vi "Red Pitaya Control.vi"(8 "Error In":errorcluster, 10 "Server port":u16=1002, 11 "Server address":string="192.168.1.100") -> (0 "Error Out":errorcluster)   [LabVIEW 2016]
uses:
  Mode.ctl
  Red Pitaya Parameters.ctl
  Waform generation/I-V parameters.ctl
  RP Command.ctl
  RP Config Offsets.ctl
  RP Write Command TCP.vi
  RP Read Temperature TCP.vi
  RP Read Status TCP.vi
  RP Read Subset TCP.vi
panel:
  in  "I-V parameters":T1={"Start magnitude"=0.001, "Magnitude increment"=0.001, "Number of pulses"=7, "Baseline length"=480, "Ramp length"=32, "Top  length"=480, "Threshold "=0.0001, "Processing delay"=255, "Valhalla range"=0.01, "Interpolation"=64} {"Valhalla range" format="%#_6pA"; "Processing delay" format="%dpts"; "Threshold" format="%#_6pV"; "Top  length" format="%dpts"; "Ramp length" format="%dpts"; "Baseline length" format="%dpts"; "Magnitude increment" format="%#_6pA"; "Start magnitude" format="%#_6pA"}
  in  "no bram":bool
  out "Output Waveform":i16[](graph)
  in  "Write waveform":bool
  in  "Controls":enum32{"Basic", "Advanced"}(tab)
  out "X&Y":cluster{i32, i32}(graph)
  in  "Parameters":T2={"Ranges"=[0.01, 0.01], "Output frequency 1"=15625000.0, "Output frequency 2"=50000.0, "Pre-trigger samples"=600000, "Post-trigger samples"=11534336, "Desimation rate"=1, "Delayed start"=571428} {"Delayed start" format="0x%x (%d)"; "Post-trigger samples" format="0x%x (%d)"; "Pre-trigger samples" format="0x%x (%d)"; "Output frequency 2" format="%#_6p"; "Output frequency 1" format="%#_6p"; "Ranges" format="%#_12p"}
  out "CPU Temperature":dbl(slide)=48.847186279148 scale=0.0..100.0
  out "Y":i32=1717987 format="0x%x (%d)"
  out "X":i32=1717987 format="0x%x (%d)"
  in  "Read XY":bool
  in  "Trigger pos acuracy":i32=1
  in  "Signal bits":i32=14
  in  "Read Temperature":bool
  in  "Read trigger":bool=TRUE
  in  "Start server":bool
  in  "FPGA Logic":enum16{"Digitizer", "Fast Digitizer"}(ring)
  in  "Auto-save file":bool
  in  "Samples to read":u64=67108864 format="0x%x (%d)"
  in  "Record":bool
  out "Server  output":string
  out "Temperature Chart":dbl(graph)=48.847186279148
  out "bytes written":i32=8
  in  "Status":bool
  out "Status response":u32=4294967115 format="0x%x (%d)"
  out "element":u32
  in  "Status offset":u64=12
  out "Record start pos":u32=20519343
  out "x-y":u32=181
  out "Phase increment 2":u64=1717987
  out "Phase increment 1":u64=1717987 format="0x%x (%d)"
  in  "Process Stop Button":bool
  in  "Read":bool
  in  "Baseline start":u16=255
  in  "Send \"Connect client\"":bool=TRUE
  out "sts bits":u32=3 format="%07b"
  in  "Read subset":bool
  out "Data File  Path":path=path "C:/Data/January_2017/011017/rp194452_011017.tdms"
  out "Trigger state":bool
  in  "Trigger":bool
  in  "Arm":bool
  out "Phase  Graph":u32[](graph)
  in  "Mode":T3=enum."Current-Voltage"
  out "Waveform Graph":sgl[][](graph)
  in  "Stop Server":bool
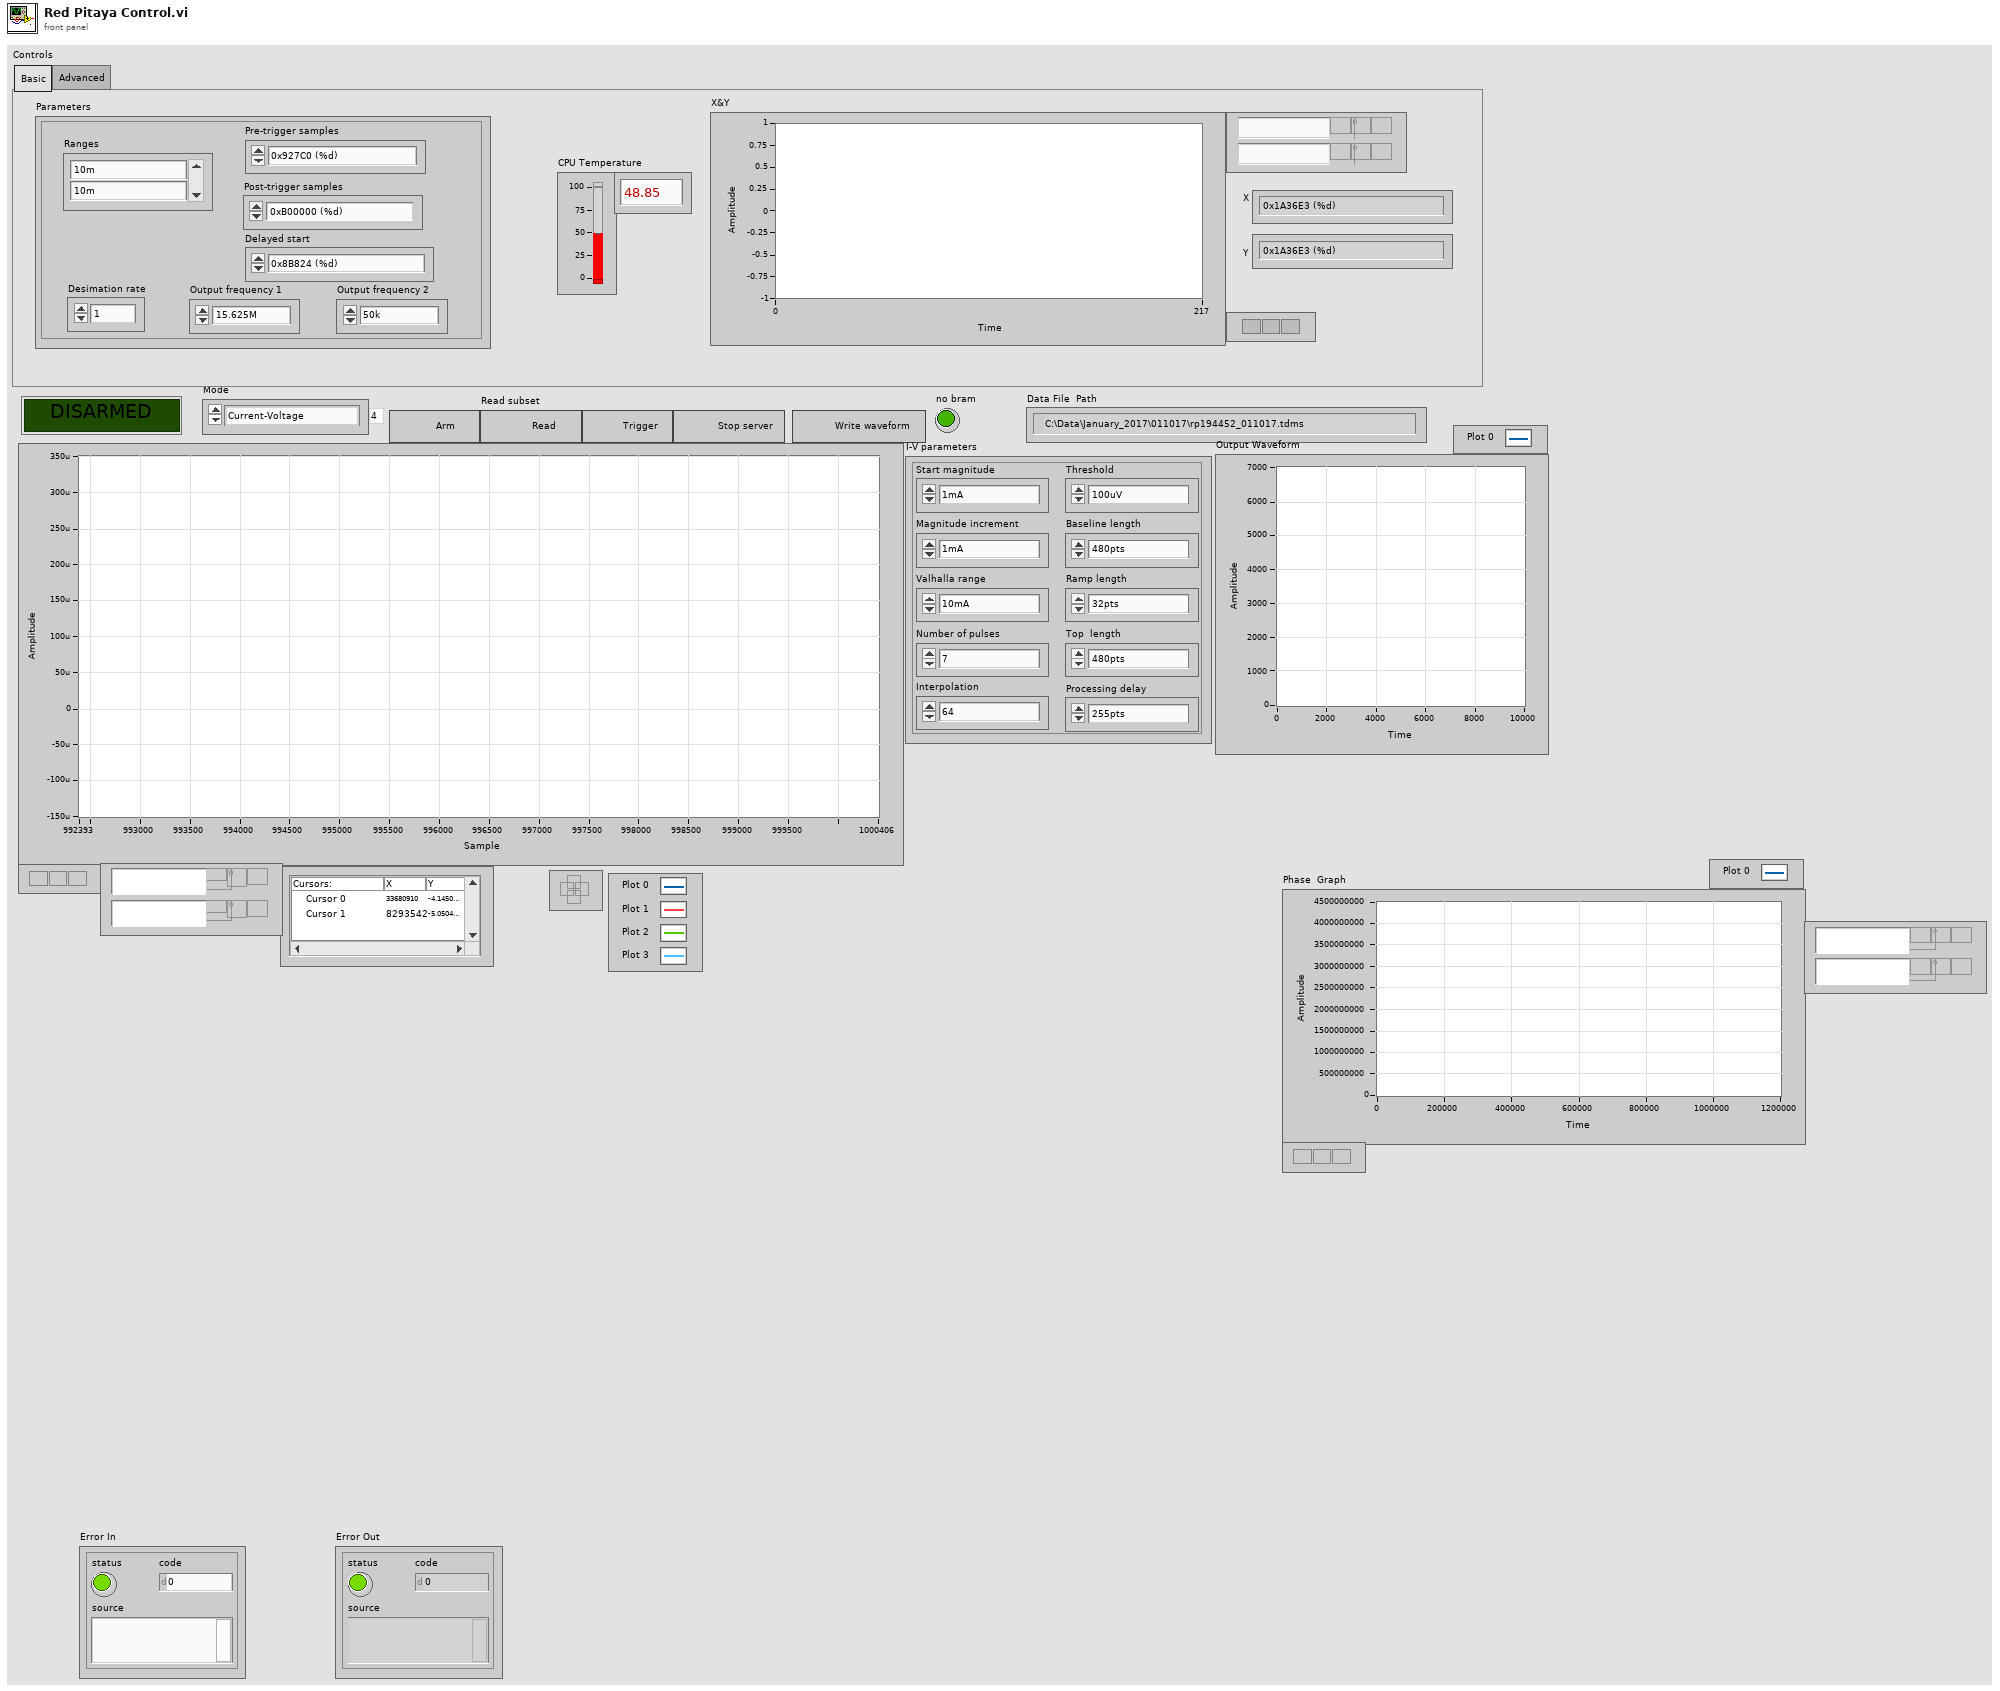
[diagram p1: front panel]
types:
  T1 = typedef "I-V parameters.ctl" = cluster{"Start magnitude":dbl, "Magnitude increment":dbl, "Number of pulses":i32, "Baseline length":i32, "Ramp length":i32, "Top  length":i32, "Threshold ":dbl, "Processing delay":u16, "Valhalla range":dbl, "Interpolation":i32}
  T2 = typedef "Red Pitaya Parameters.ctl" = cluster{"Ranges":dbl[], "Output frequency 1":dbl, "Output frequency 2":dbl, "Pre-trigger samples":i32, "Post-trigger samples":u64, "Desimation rate":u64, "Delayed start":u64}
  T3 = typedef "Mode.ctl" = enum16{"Filter", "Lockin test", "Snapshot test", "Digitizer", "Current-Voltage"}
  T4 = typedef "RP Command.ctl" = enum16{"Reset", "Read IDN", "Stop server", "Get status", "Get temperature", "Connect client", "Arm", "Software trigger", "Get whole buffer", "Get chunk", "System call", "Get config", "Set config", "Recieve data", "Recieve Calibartion", "Transmit data"}
  T5 = typedef "RP Config Offsets.ctl" = u16
  T6 = typedef "Waveform parameters.ctl" = cluster{"Start magnitude":dbl, "Magnitude increment":dbl, "Number of pulses":i32, "Baseline length":i32, "Ramp length":i32, "Top  length":i32, "Threshold ":i32, "Processing delay":u16}
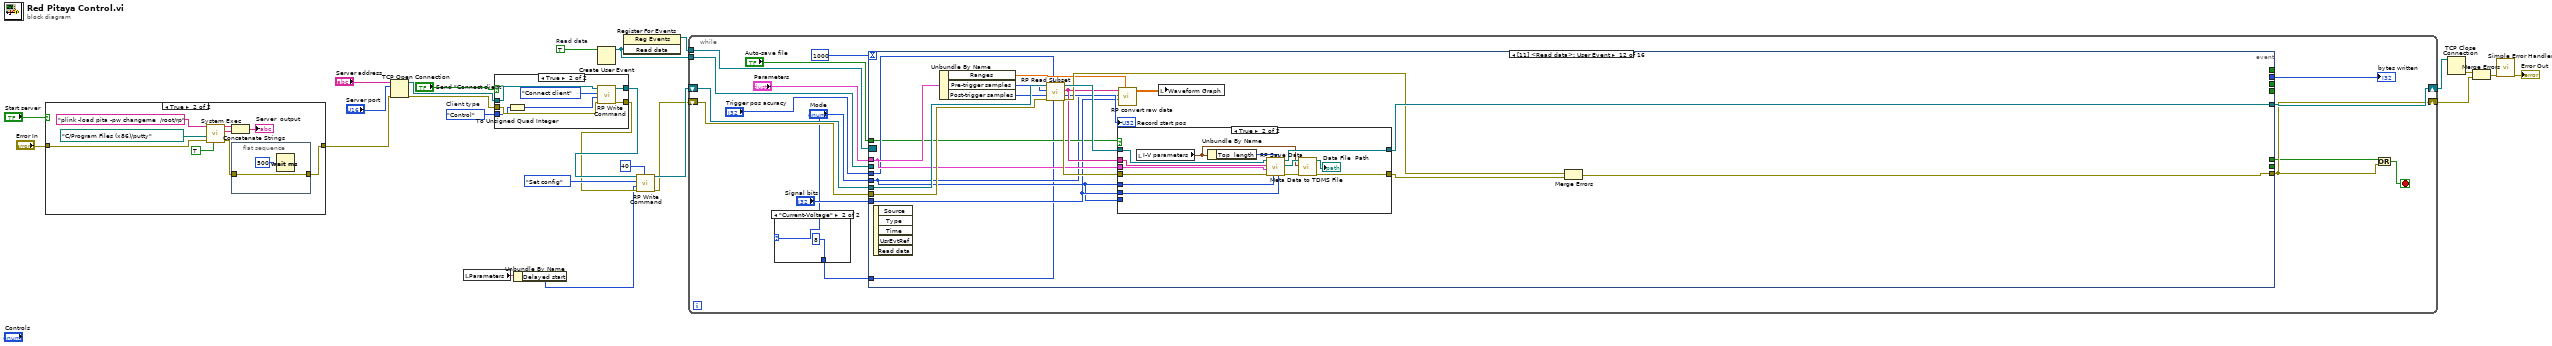
[diagram p0: block diagram]
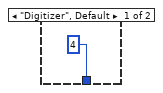
[diagram p4: hidden frame]
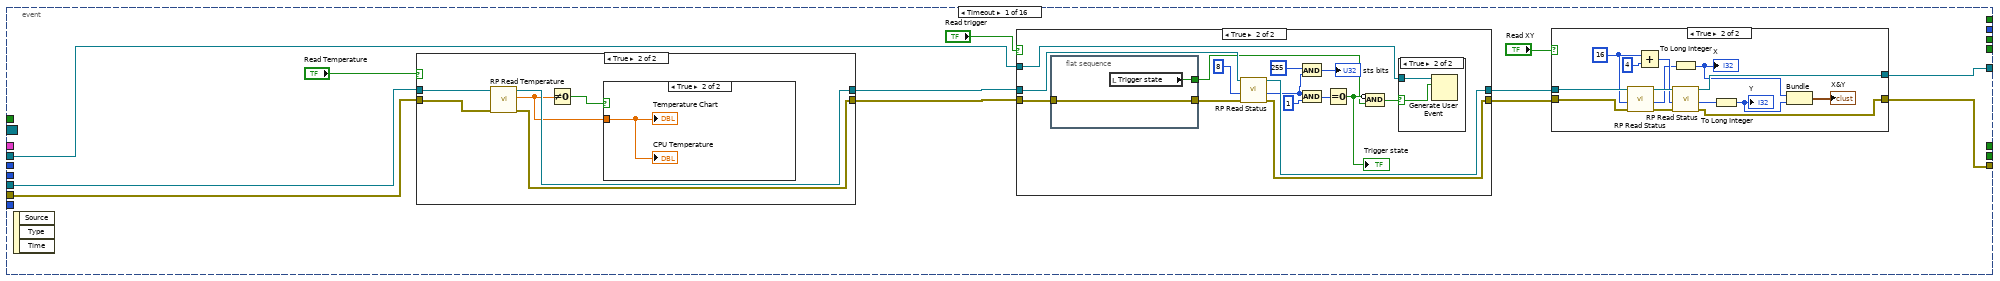
[diagram p5: hidden frame]
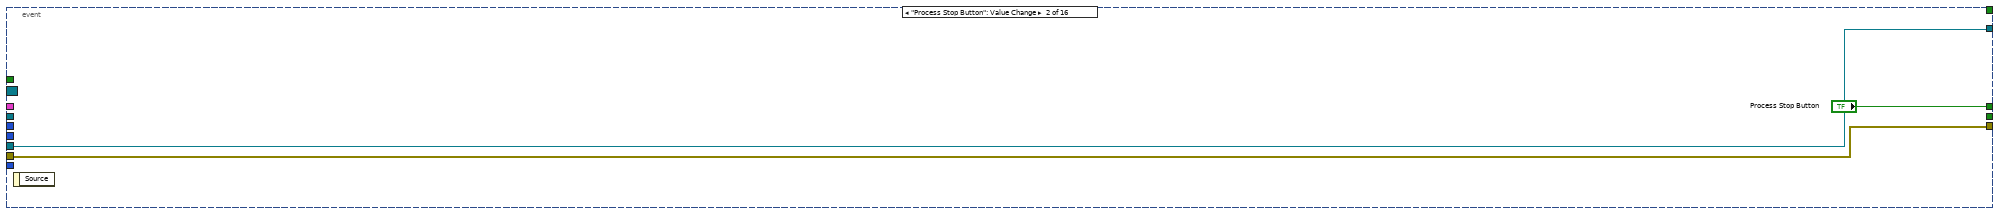
[diagram p11: hidden frame]
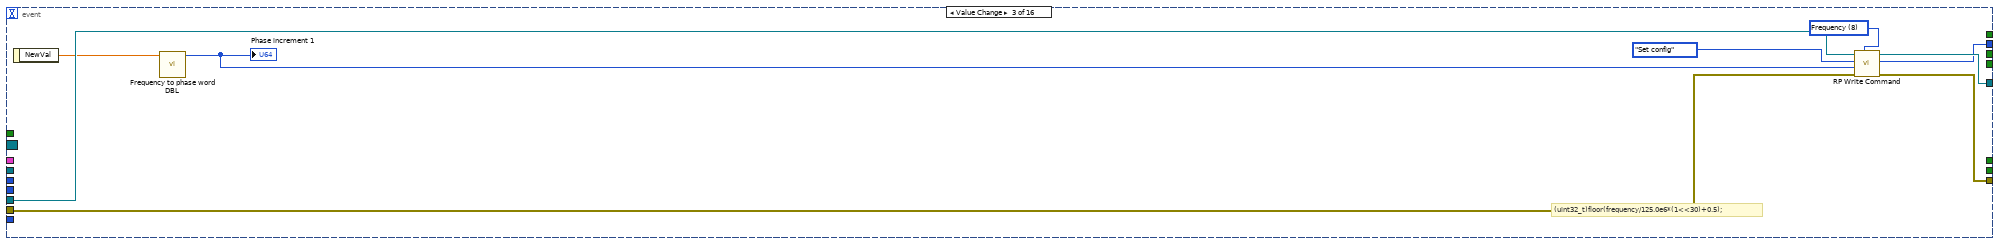
[diagram p12: hidden frame]
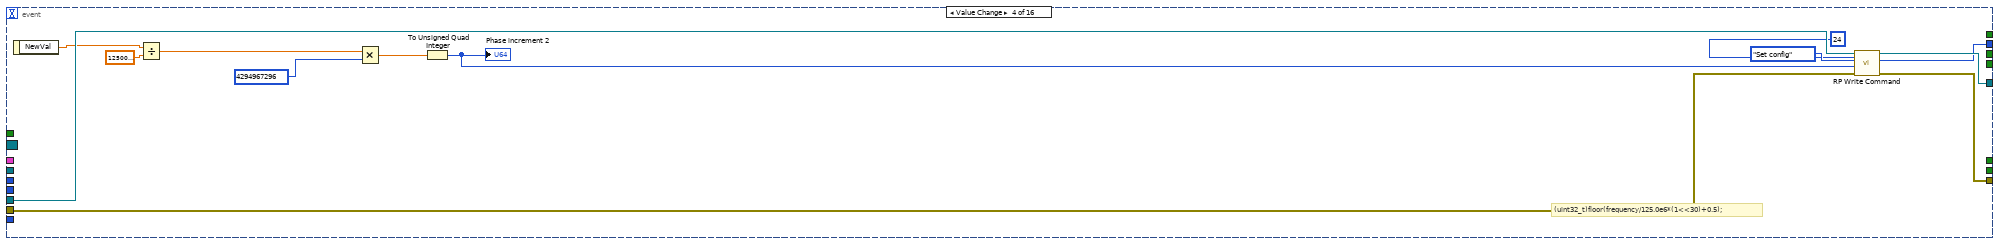
[diagram p13: hidden frame]
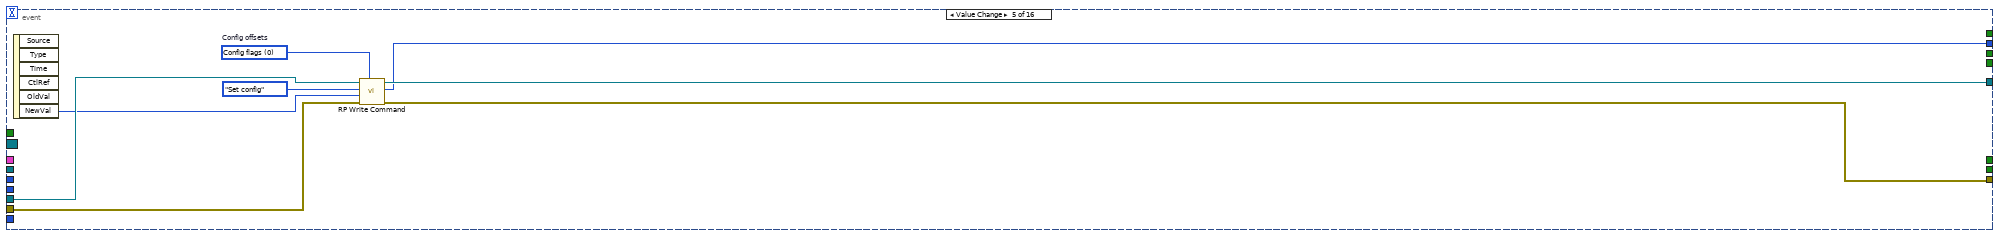
[diagram p14: hidden frame]
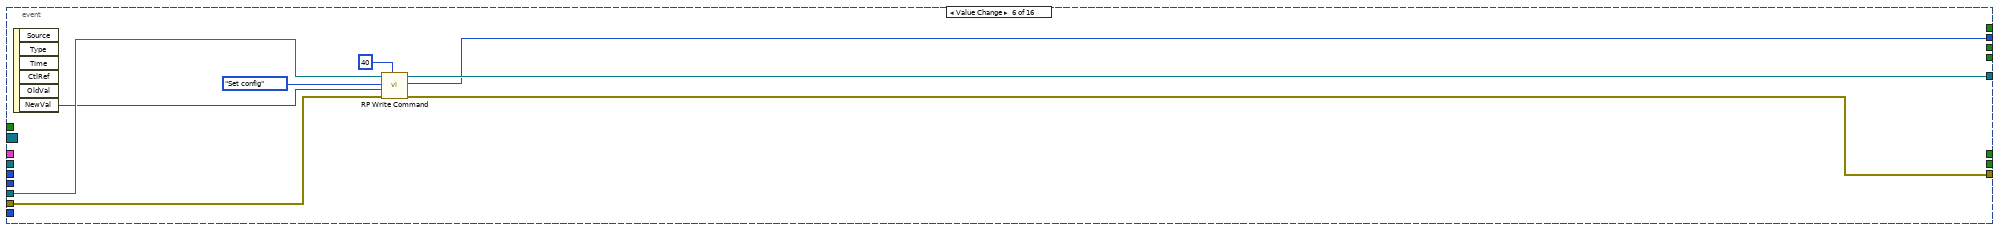
[diagram p15: hidden frame]
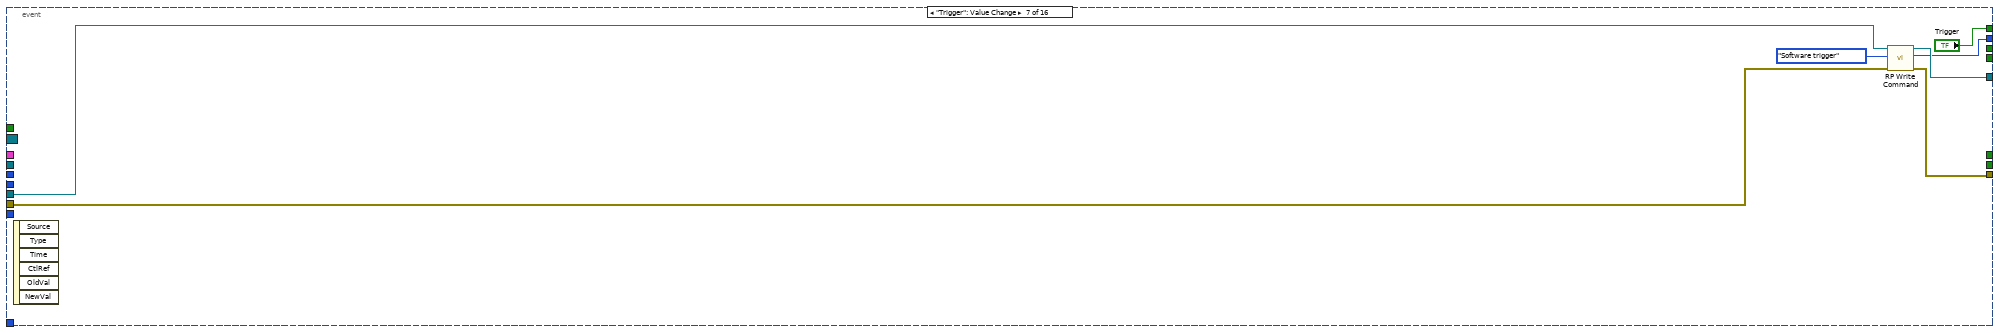
[diagram p16: hidden frame]
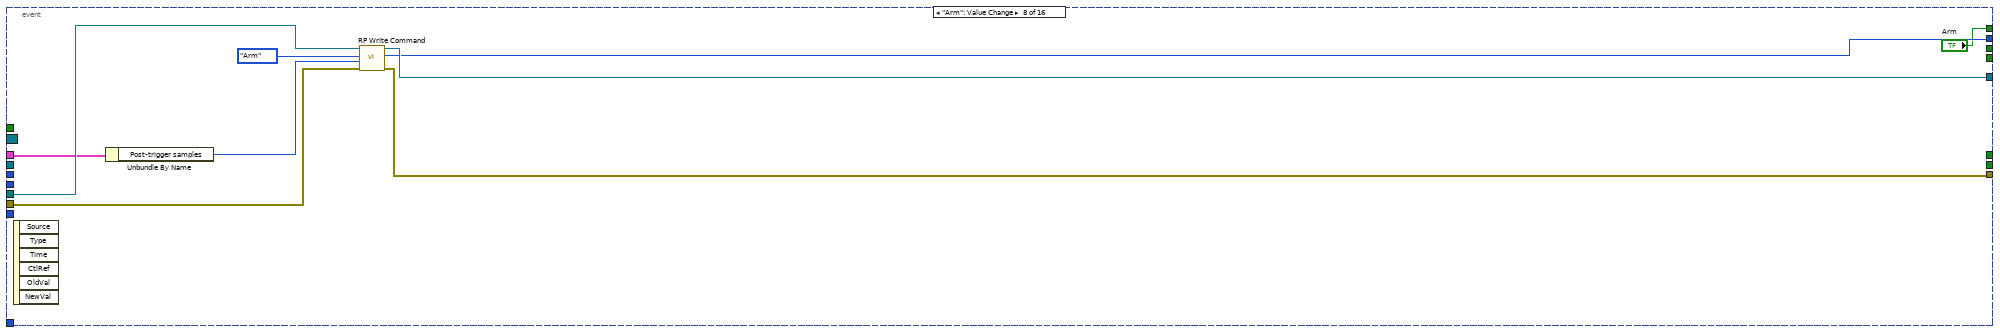
[diagram p17: hidden frame]
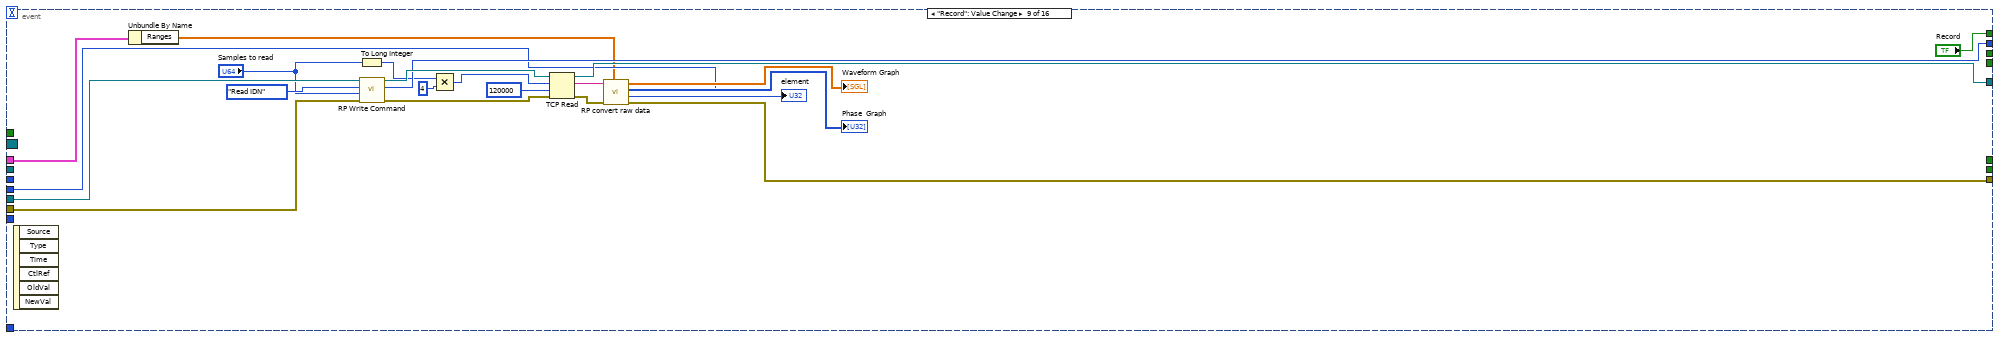
[diagram p18: hidden frame]
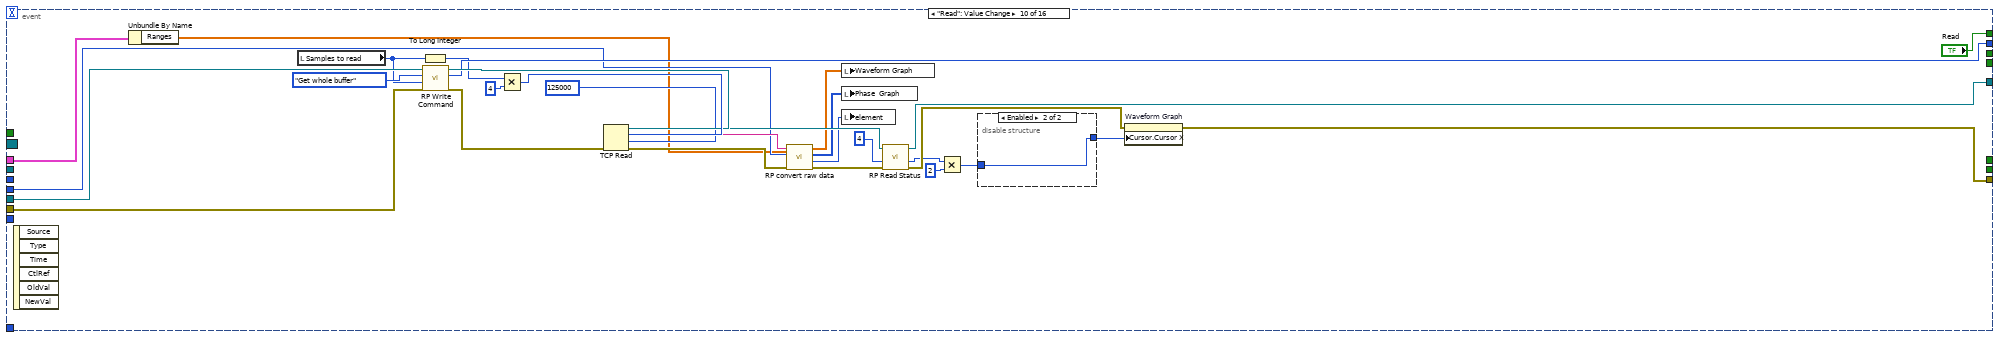
[diagram p19: hidden frame]
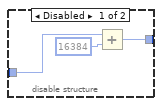
[diagram p20: hidden frame]
diagram:
  w9 = enum16{"Control", "Reciever", "Transmitter"}."Control"  # Client type
  w15 = TRUE  # Read data
  n1 = case shown="True" "Start server" {
    tunnel: [w26 w27] -> w17
    tunnel: "Error In" -> [w26 w29]
    frame False {
    }
    frame True {
      n2 = call <vilib>:"System Exec.vi"("run minimized? (F)"=TRUE, "error in (no error)"=w29, "working directory"=path "C:/Program Files (x86)/putty", "command line"="plink -load pita -pw changeme  /root/rp") -> ("error out"=w28:errorcluster, "standard error"=w31:string, "standard output"=w35:string)  [unwired: 4 in, 1 out]
      n3 = Concatenate Strings(w35, w31) -> (→"Server  output":string)
      n4 = flat-sequence {
        tunnel: w28 -> [w37]
        tunnel: [w37] -> w27
        frame #0 {
          n5 = Wait (ms)(milliseconds to wait=u32 500) -> ()  [unwired: 1 out]
        }
      }
    }
  }
  n6 = TCP Open Connection(address="Server address", remote port or service name="Server port", error in (no error)=w17) -> (connection ID=w10:refnum<k5>, error out=w11:errorcluster)  [unwired: 2 in]
  n7 = local read "Parameters"() -> (w2:T2)
  n8 = case shown="True" "Send \"Connect client\"" {
    tunnel: w11 -> [w38 w46]
    tunnel: w10 -> [w39 w45]
    tunnel: w9 -> [_ w43]
    tunnel: [w39 w41] -> w6
    tunnel: [w38 w40] -> w4
    frame False {
    }
    frame True {
      n9 = To Unsigned Quad Integer(1:w43) -> (0:w42:u64)
      n10 = call-poly "RP Write Command.vi"("Error In"=w46, "Command payload"=w42, "Command number"=RP_Command."Connect client", "connection ID"=w45) -> ("Error Out"=w40:errorcluster, "connection ID out"=w41:refnum<k5>)  [unwired: 5 in, 1 out]
    }
  }
  n11 = Unbundle By Name(w2) -> ("Delayed start"=w1:u64)
  n12 = Create User Event(user event datatype=w15) -> (user event=w13:refnum<user-event>)  [unwired: 1 in, 1 out]
  n13 = register-events(w13) -> (reference out=w14:refnum<event-registration>)  [unwired: 2 in, 1 out]
  n14 = call-poly "RP Write Command.vi"("Config offset"=u64 40, "Error In"=w4, "Command payload"=w1, "Command number"=RP_Command."Set config", "connection ID"=w6) -> ("Error Out"=w3:errorcluster, "connection ID out"=w5:refnum<k5>)  [unwired: 4 in, 1 out]
  n15 = while {
    shift-right: [w60] -> w21
    shift-left: w5 -> [w61]
    shift-right: [w58] -> w20
    shift-left: w3 -> [w62]
    tunnel: w14 -> [w50]
    tunnel: w13 -> [w49]
    stop <- w56 stop-if-true
    n16 = case shown="\"Current-Voltage\"" "Mode" {
      tunnel: [4 8] -> w47
      frame "Digitizer", Default {
      }
      frame "Current-Voltage" {
      }
    }
    n17 = event shown="[11] <Read data>: User Event" {
      selector: w50 -> [_ _ _ _ _ _ _ _ _ _ _ _ _ _ _ _]
      dyn-events: _ -> [_ _ _ _ _ _ _ _ _ _ _ _ _ _ _ _]
      timeout: 1000 -> [_ _ _ _ _ _ _ _ _ _ _ _ _ _ _ _]
      tunnel: w62 -> [w74 w124 w134 w143 w155 w163 w170 w179 w194 w226 w244 w263 w283 w295 w302 w308]
      tunnel: w61 -> [w75 w123 w133 w142 w154 w162 w169 w178 w197 w229 w246 w262 w284 w294 w300 w304]
      tunnel: [w67 w124 w130 w138 w151 w159 w166 w175 w185 w223 w243 w266 w282 w290 w299 w307] -> w58
      tunnel: [w68 w123 w131 w139 w152 w160 w167 w176 w199 w219 w245 w264 w284 w289 w298 w305] -> w60
      tunnel: [_ "Process Stop Button" _ _ _ _ _ _ _ _ _ _ _ _ "Stop Server" _] -> w57
      tunnel: [_ _ _ _ _ _ _ _ _ _ _ _ _ _ _ "Status"] -> _
      tunnel: [_ _ w129 w137 w150 w158 w165 w174 w192 w224 _ _ _ w288 w297 _] -> w59
      tunnel: [_ _ _ _ _ _ "Trigger" "Arm" "Record" "Read" _ _ _ _ _ _] -> _
      tunnel: "Mode" -> [_ _ _ _ _ _ _ _ w182 w204 _ w249 _ _ _ _]
      tunnel: "Parameters" -> [_ _ _ _ _ _ _ w172 w181 w203 w238 w257 _ _ _ _]
      tunnel: "Signal bits" -> [_ _ _ _ _ _ _ _ _ _ _ w254 _ _ _ _]
      tunnel: "Trigger pos acuracy" -> [_ _ _ _ _ _ _ _ _ _ _ w255 _ _ _ _]
      tunnel: [_ _ _ _ _ _ _ _ _ _ "Write waveform" _ _ _ _ _] -> _
      tunnel: "Auto-save file" -> [_ _ _ _ _ _ _ _ _ _ _ w252 _ _ _ _]
      tunnel: [_ _ _ _ _ _ _ _ _ _ _ _ "Read subset" _ _ _] -> _
      tunnel: w49 -> [w65 _ _ _ _ _ _ _ _ _ _ _ w286 _ _ _]
      tunnel: w47 -> [_ _ _ _ _ _ _ _ _ _ _ w248 _ _ _ _]
      event Timeout {
        n18 = event-data() -> ()  [unwired: 1 in, 3 out]
        n19 = case shown="True" "Read Temperature" {
          tunnel: w75 -> [w115 w120]
          tunnel: w74 -> [w114 w116]
          tunnel: [w115 w119] -> w72
          tunnel: [w114 w117] -> w71
          frame False {
          }
          frame True {
            n20 = call-poly "RP Read Temperature.vi"("Error In"=w116, "connection ID"=w120) -> ("error out"=w117:errorcluster, "Thermometer"=w118:dbl, "connection ID out"=w119:refnum<k5>)  [unwired: 7 in]
            n21 = Not Equal To 0?(x=w118) -> (x != 0?=w121:bool)
            n22 = case shown="True" w121 {
              tunnel: w118 -> [_ w122]
              frame False {
              }
              frame True {
                "CPU Temperature" <- w122
                "Temperature Chart" <- w122
              }
            }
          }
        }
        n23 = case shown="True" "Read trigger" {
          tunnel: w72 -> [w93 w109]
          tunnel: w71 -> [w94 w103]
          tunnel: [w94 w106] -> w70
          tunnel: [w93 w104] -> w69
          tunnel: w65 -> [_ w98]
          frame False {
          }
          frame True {
            n24 = flat-sequence {
              tunnel: w103 -> [w113]
              tunnel: [w113] -> w102
              tunnel: [w112] -> w100
              frame #0 {
                n25 = local read "Trigger state"() -> (w112:bool)
              }
            }
            n26 = call-poly "RP Read Status.vi"("Error In"=w102, "Status offset"=u64 8, "connection ID"=w109) -> ("Error Out"=w106:errorcluster, "Status response"=w97:u32, "connection ID out"=w104:refnum<k5>)  [unwired: 6 in]
            n27 = And(x=u32 255 ("y"), y=w97) -> (x .and. y?=→"sts bits":u32)
            n28 = And(x=w97, y=u32 1) -> (x .and. y?=w105:u32)
            n29 = Equal To 0?(x=w105) -> (x = 0?=w101:bool)
            "Trigger state" <- w101
            n30 = Compound Arithmetic op=AND(invert w101, w100) -> (w99:bool)
            n31 = case shown="True" w99 {
              selector: w99 -> [_ w110]
              tunnel: w98 -> [_ w111]
              frame False {
              }
              frame True {
                n32 = Generate User Event(user event=w111, event data cluster=w110) -> ()  [unwired: 2 in, 2 out]
              }
            }
          }
        }
        n33 = case shown="True" "Read XY" {
          tunnel: w69 -> [w77 w91]
          tunnel: w70 -> [w78 w92]
          tunnel: [w78 w89] -> w67
          tunnel: [w77 w87] -> w68
          frame False {
          }
          frame True {
            w86 = u64 16 ("Status offset")
            n34 = call-poly "RP Read Status.vi"("Error In"=w92, "Status offset"=w86, "connection ID"=w91) -> ("Error Out"=w90:errorcluster, "Status response"=w83:u32, "connection ID out"=w88:refnum<k5>)  [unwired: 6 in]
            n35 = Add(x=w86, y=u64 4) -> (x+y=w84:u64)
            n36 = To Long Integer(number=w83) -> (32bit integer=w81:i32)
            "X" <- w81
            n37 = call-poly "RP Read Status.vi"("Error In"=w90, "Status offset"=w84, "connection ID"=w88) -> ("Error Out"=w89:errorcluster, "Status response"=w82:u32, "connection ID out"=w87:refnum<k5>)  [unwired: 6 in]
            n38 = To Long Integer(number=w82) -> (32bit integer=w80:i32)
            "Y" <- w80
            n39 = Bundle(w81, w80) -> (→"X&Y":cluster{i32, i32})  [unwired: 1 in]
          }
        }
      }
      event "Process Stop Button": Value Change {
        n40 = event-data() -> ()  [unwired: 1 in, 1 out]
      }
      event Value Change {
        w126 = T5 8 items=["Config flags"=0, "Record length"=4, "Frequency"=8, "Decimation"=12, "LED"=16, "DDS delay"=28] ("Config offset")
        # "(uint32_t)floor(frequency/125.0e6*(1<<30)+0.5);"
        n41 = event-data() -> ("NewVal"=w128:dbl)  [unwired: 1 in]
        n42 = call "Frequency to phase word DBL.vi"("Frequency"=w128) -> ("Phase word"=w127:u64)  [unwired: 9 in, 1 out]
        "Phase increment 1" <- w127
        n43 = call-poly "RP Write Command.vi"("Config offset"=w126, "Error In"=w134, "Command payload"=w127, "Command number"=RP_Command."Set config", "connection ID"=w133) -> ("Error Out"=w130:errorcluster, "bytes written"=w129:i32, "connection ID out"=w131:refnum<k5>)  [unwired: 4 in]
      }
      event Value Change {
        # "(uint32_t)floor(frequency/125.0e6*(1<<30)+0.5);"
        n44 = event-data() -> ("NewVal"=w135:dbl)  [unwired: 1 in]
        n45 = Divide(x=w135, y=125000000.0) -> (x/y=w145:dbl)
        n46 = Multiply(x=w145, y=i64 4294967296) -> (x*y=w144:dbl)
        n47 = To Unsigned Quad Integer(1:w144) -> (0:w140:u64)
        "Phase increment 2" <- w140
        n48 = call-poly "RP Write Command.vi"("Config offset"=u64 24, "Error In"=w143, "Command payload"=w140, "Command number"=RP_Command."Set config", "connection ID"=w142) -> ("Error Out"=w138:errorcluster, "bytes written"=w137:i32, "connection ID out"=w139:refnum<k5>)  [unwired: 4 in]
      }
      event Value Change {
        w148 = T5 0 items=["Config flags"=0, "Record length"=4, "Frequency"=8, "Decimation"=12, "LED"=16, "DDS delay"=28]  # Config offsets
        n49 = event-data() -> ("NewVal"=w149:u64)  [unwired: 1 in, 5 out]
        n50 = call-poly "RP Write Command.vi"("Config offset"=w148, "Error In"=w155, "Command payload"=w149, "Command number"=RP_Command."Set config", "connection ID"=w154) -> ("Error Out"=w151:errorcluster, "bytes written"=w150:i32, "connection ID out"=w152:refnum<k5>)  [unwired: 4 in]
      }
      event Value Change {
        n51 = event-data() -> ("NewVal"=w157:u64)  [unwired: 1 in, 5 out]
        n52 = call-poly "RP Write Command.vi"("Config offset"=u64 40, "Error In"=w163, "Command payload"=w157, "Command number"=RP_Command."Set config", "connection ID"=w162) -> ("Error Out"=w159:errorcluster, "bytes written"=w158:i32, "connection ID out"=w160:refnum<k5>)  [unwired: 4 in]
      }
      event "Trigger": Value Change {
        n53 = event-data() -> ()  [unwired: 1 in, 6 out]
        n54 = call-poly "RP Write Command.vi"("Error In"=w170, "Command number"=RP_Command."Software trigger", "connection ID"=w169) -> ("Error Out"=w166:errorcluster, "bytes written"=w165:i32, "connection ID out"=w167:refnum<k5>)  [unwired: 6 in]
      }
      event "Arm": Value Change {
        n55 = event-data() -> ()  [unwired: 1 in, 6 out]
        n56 = Unbundle By Name(w172) -> ("Post-trigger samples"=w171:u64)
        n57 = call-poly "RP Write Command.vi"("Error In"=w179, "Command payload"=w171, "Command number"=RP_Command."Arm", "connection ID"=w178) -> ("Error Out"=w175:errorcluster, "bytes written"=w174:i32, "connection ID out"=w176:refnum<k5>)  [unwired: 5 in]
      }
      event "Record": Value Change {
        n58 = event-data() -> ()  [unwired: 1 in, 6 out]
        n59 = Unbundle By Name(w181) -> ("Ranges"=w180:dbl[])
        n60 = To Long Integer(number="Samples to read") -> (32bit integer=w191:i32)
        n61 = call-poly "RP Write Command.vi"("Error In"=w194, "Command payload"="Samples to read", "Command number"=RP_Command."Read IDN", "connection ID"=w197) -> ("Error Out"=w193:errorcluster, "bytes written"=w192:i32, "connection ID out"=w195:refnum<k5>)  [unwired: 5 in]
        n62 = Multiply(x=w191, y=4) -> (x*y=w198:i32)
        n63 = TCP Read(connection ID=w195, bytes to read=w198, error in (no error)=w193, 9:120000 ("timeout ms (25000)")) -> (connection ID out=w199:refnum<k5>, data out=w188:string, error out=w186:errorcluster)  [unwired: 1 in]
        n64 = call "RP convert raw data.vi"("Max Volts"=w180, "Error In"=w186, "Format"=w182, "data stream"=w188) -> ("Error Out"=w185:errorcluster, "element"=→"element":u32, "phase out"=→"Phase  Graph":u32[], "data out"=→"Waveform Graph":sgl[][])  [unwired: 4 in]
      }
      event "Read": Value Change {
        n65 = event-data() -> ()  [unwired: 1 in, 6 out]
        n66 = Unbundle By Name(w203) -> ("Ranges"=w202:dbl[])
        n67 = local read "Samples to read"() -> (w218:u64)
        n68 = To Long Integer(number=w218) -> (32bit integer=w221:i32)
        n69 = call-poly "RP Write Command.vi"("Error In"=w226, "Command payload"=w218, "Command number"=RP_Command."Get whole buffer", "connection ID"=w229) -> ("Error Out"=w225:errorcluster, "bytes written"=w224:i32, "connection ID out"=w227:refnum<k5>)  [unwired: 5 in]
        n70 = Multiply(x=w221, y=4) -> (x*y=w230:i32)
        n71 = TCP Read(connection ID=w227, bytes to read=w230, error in (no error)=w225, 9:125000 ("timeout ms (25000)")) -> (connection ID out=w220:refnum<k5>, data out=w216:string, error out=w206:errorcluster)  [unwired: 1 in]
        n72 = call "RP convert raw data.vi"("Max Volts"=w202, "Error In"=w206, "Format"=w204, "data stream"=w216) -> ("Error Out"=w205:errorcluster, "element"=w213:u32, "phase out"=w214:u32[], "data out"=w215:sgl[][])  [unwired: 4 in]
        n73 = local write "Waveform Graph"(w215) -> ()
        n74 = local write "Phase  Graph"(w214) -> ()
        n75 = local write "element"(w213) -> ()
        n76 = call-poly "RP Read Status.vi"("Error In"=w205, "Status offset"=u64 4, "connection ID"=w220) -> ("Error Out"=w211:errorcluster, "Status response"=w210:u32, "connection ID out"=w219:refnum<k5>)  [unwired: 6 in]
        n77 = Multiply(x=w210, y=u32 2) -> (x*y=w208:u32)
        n78 = disable-structure shown="Enabled" {
          disable-tunnel: w208 -> [w234 w235]
          disable-tunnel: [w232 w235] -> w207
          frame Disabled {
            n79 = Add(x=w234, y=16384) -> (x+y=w232:u32)
          }
          frame Enabled {
          }
        }
        n80 = property on="Waveform Graph" class="WFGraph (strict)"(error in=w211, "Cursor.Cursor X"=w207) -> (error out=w223:errorcluster)  [unwired: 1 in, 1 out]
      }
      event "Write waveform": Value Change {
        n81 = event-data() -> ()  [unwired: 1 in, 6 out]
        n82 = Unbundle By Name(w238) -> ("Ranges"=w237:dbl[])
        n83 = Index Array(array=w237) -> (element=w236:dbl)  [unwired: 1 in]
        n84 = call "I-V to Waveform parameters.vi"("Input range"=w236, "I-V parameters"="I-V parameters") -> ("Waveform parameters out"=w239:T6)  [unwired: 9 in]
        n85 = call "RP IV pattern write.vi"("no bram"="no bram", "Error In"=w244, "Waveform parameters"=w239, "connection ID"=w246) -> ("Error Out"=w243:errorcluster, "connection ID out"=w245:refnum<k5>, "Waveform Graph"=→"Output Waveform":i16[])  [unwired: 5 in]
      }
      event User Event {
        n86 = event-data() -> ()  [unwired: 1 in, 5 out]
        n87 = Unbundle By Name(w257) -> ("Ranges"=w256:dbl[], "Pre-trigger samples"=w251:i32, "Post-trigger samples"=w250:u64)
        n88 = call-poly "RP Read Subset.vi"("Bytes per sample"=w248, "Samples per trigger increment"=w255, "Error In"=w263, "Post-trigger samples"=w250, "Pre-trigger samples"=w251, "connection ID"=w262) -> ("Error Out"=w260:errorcluster, "Record start pos"=→"Record start pos":u32, "Data stream"=w259:string, "connection ID out"=w261:refnum<k5>)  [unwired: 2 in]
        n89 = case shown="True" w252 {
          tunnel: w260 -> [w268 w276]
          tunnel: w259 -> [_ w279]
          tunnel: [w268 w271] -> w265
          tunnel: w261 -> [w267 w281]
          tunnel: [w267 w277] -> w264
          tunnel: w257 -> [_ w280]
          tunnel: w249 -> [_ w278]
          tunnel: w254 -> [_ w275]
          tunnel: w249 -> [_ _]
          frame False {
          }
          frame True {
            n90 = local read "I-V parameters"() -> (w270:T1)
            n91 = Unbundle By Name(w270) -> ("Top  length"=w269:i32)
            n92 = call "RP Save Data.vi"("Signal bits"=w275, "I-V avg"=w269, "Mode"=w278, "Error In"=w276, "Parameters"=w280, "Data stream"=w279, "connection ID"=w281) -> ("Error Out"=w272:errorcluster, "Data File  Path"=w274:path, "connection ID out"=w277:refnum<k5>)  [unwired: 1 in, 1 out]
            n93 = call "Meta Data to TDMS File.vi"("Error In"=w272, "Value"=w270, "File Path"=w274) -> ("Error Out"=w271:errorcluster, "File Path out"=→"Data File  Path":path)  [unwired: 7 in]
          }
        }
        n94 = call "RP convert raw data.vi"("Max Volts"=w256, "Signal bits"=w254, "Format"=w249, "data stream"=w259) -> ("data out"=w253:sgl[][])  [unwired: 4 in, 3 out]
        n95 = local write "Waveform Graph"(w253) -> ()
        n96 = Merge Errors(w260, w265) -> (w266:errorcluster)
      }
      event "Read subset": Value Change {
        n97 = event-data() -> ()  [unwired: 1 in, 6 out]
        n98 = Generate User Event(user event=w286, event data cluster=TRUE, error in=w283) -> (error out=w282:errorcluster)  [unwired: 1 in, 1 out]
      }
      event "FPGA Logic": Value Change {
        n99 = event-data() -> ()  [unwired: 1 in, 6 out]
        n100 = To Unsigned Quad Integer(1:"FPGA Logic") -> (0:w292:u64)
        n101 = call-poly "RP Write Command.vi"("Error In"=w295, "Command payload"=w292, "Command number"=RP_Command."System call", "connection ID"=w294) -> ("Error Out"=w290:errorcluster, "bytes written"=w288:i32, "connection ID out"=w289:refnum<k5>)  [unwired: 5 in]
      }
      event "Stop Server": Value Change {
        n102 = event-data() -> ()  [unwired: 1 in, 6 out]
        n103 = call-poly "RP Write Command.vi"("Error In"=w302, "Command number"=RP_Command."Stop server", "connection ID"=w300) -> ("Error Out"=w299:errorcluster, "bytes written"=w297:i32, "connection ID out"=w298:refnum<k5>)  [unwired: 6 in]
      }
      event "Status": Value Change {
        (unwired) u64 12 ("Status offset")
        n104 = event-data() -> ()  [unwired: 1 in, 6 out]
        n105 = local read "element"() -> (w310:u32)
        n106 = call-poly "RP Read Status.vi"("Error In"=w308, "Status offset"="Status offset", "connection ID"=w304) -> ("Error Out"=w307:errorcluster, "Status response"=w306:u32, "connection ID out"=w305:refnum<k5>)  [unwired: 6 in]
        "Status response" <- w306
        n107 = Subtract(x=w310, y=w306) -> (x-y=→"x-y":u32)
      }
    }
    "bytes written" <- w59
    n108 = Or(x=w57, y=w58) -> (x .or. y?=w56:bool)
  }
  n109 = TCP Close Connection(connection ID=w21) -> (error out=w23:errorcluster)  [unwired: 2 in, 1 out]
  n110 = Merge Errors(w23, w20) -> (w22:errorcluster)
  n111 = call <vilib>:"Simple Error Handler.vi"("error in (no error)"=w22) -> ("error out"=→"Error Out":errorcluster)  [unwired: 4 in, 4 out]
